vi "scaler_digital_2channel_example.vi"() -> ()   [LabVIEW 2017]
uses:
  <vilib>/Platform/TimedLoop/XDataNode/timing_clust.ctl
  <vilib>/Platform/TimedLoop/XDataNode/nitl_modes.ctl
  <vilib>/Platform/TimedLoop/XDataNode/wakeup.ctl
  <vilib>/rvi/Emulation/niFpgaGetClockAttributes.vi
  <vilib>/rvi/Emulation/niFpgaSctlEmulationGetInTimedLoop.vi
  <vilib>/rvi/Emulation/niFpgaEmulationReportErrorSimple.vi
  <vilib>/rvi/eio/common/nirviEmuTemplateMethod_errors.vi
  <vilib>/rvi/Emulation/niFpgaProcessEmulError.vi
  <vilib>/rvi/Emulation/niFpgaCriticalErrorInLSC.vi
  <vilib>/eio/EIONode/EIONode.xnode
  <vilib>/Platform/TimedLoop/XDataNode/XDataNode.xnode
  <vilib>/Platform/TimedLoop/XDataNode/XDNodeRunTimeDep.lvlib
  lib/Scaler-EPICS/scaler.lvlib
panel:
  in  "Pulse_Scaler":bool[](array[boolean])=[FALSE]
  in  "OneShot_Scaler":bool
  in  "Enable_Scaler":bool
  in  "Gate_Scaler":bool[](array[boolean])=[FALSE, FALSE]
  out "Done_Scaler":bool
  out "Counter_Scaler":u32[](array[numeric])
  in  "PresetValues_Scaler":u32[](array[numeric])=[0, 0]
  # "This is a 2 channel digital scaler. It follows to the word the definition of the scaler in the anl website\nhttps://epics.anl.gov/bcda/synApps/std/scalerRecord.html"
  # "Optimization tip:\nMake all the arrays the same size as the number\nof channels you need implemented. Setting\nthe number of channels uses up to 45% of the \nresources. Setting to 2 uses only 23%."
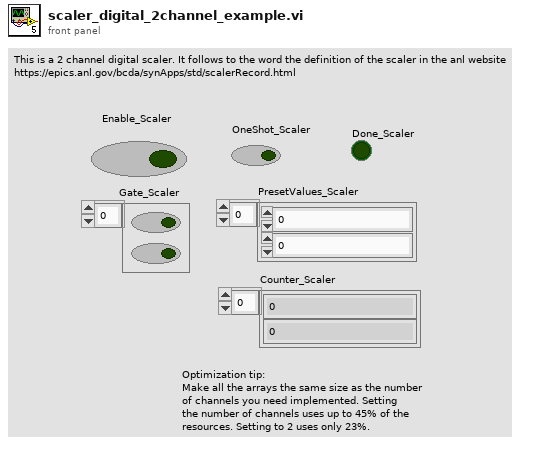
[diagram p1: front panel]
types:
  T1 = typedef "XDNodeRunTimeDep.lvlib/timing_clust.ctl" = cluster{"Expected End [f-1]":u64, "Actual End [f-1]":u64, "Finished Late? [f-1]":bool, "Expected End [i-1]":u64, "Actual End [i-1]":u64, "Finished Late? [i-1]":bool, "Expected Start [i]":u64, "Actual Start [i]":u64, "Expected Start [f]":u64, "Actual Start [f]":u64, "Source Name":string, "Structure Name":string, "Period":i64, "Deadline":i64, "Offset":i64, "Start":i64, "Priority":i32, "Timeout":i32, "Mode":T2, "Wakeup Reason":T3, "Error":errorcluster, "Source Type":string, "Secondary Source Type":string, "Global End Time":u64, "Global Start Time":u64, "Frame Duration":u64, "Iteration Duration":u64, "Assigned CPU":i32, "I/O Scan Engine Mode":u32}
  T2 = typedef "XDNodeRunTimeDep.lvlib/nitl_modes.ctl" = enum32{"No Change", "Process missed periods, maintain original phase", "Discard missed periods, maintain original phase", "Process missed periods, ignore original phase", "Discard missed periods, ignore original phase"}
  T3 = typedef "XDNodeRunTimeDep.lvlib/wakeup.ctl" = enum32{"Normal", "Aborted", "Asynchronous wakeup", "Timing source error", "Timed loop error", "Timeout"}
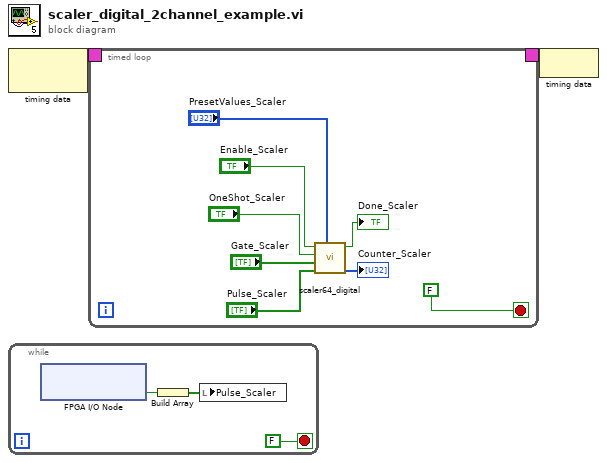
[diagram p0: block diagram]
diagram:
  n1 = node-c288() -> (w2:T1)  [unwired: 1 in]
  n2 = while {
    stop <- FALSE stop-if-true
    n3 = xnode "FPGA I/O Node"() -> ("Mod2/DIO0"=w5:bool)  [unwired: 1 in, 1 out]
    n4 = Build Array(w5) -> (w4:bool[])
    n5 = local write "Pulse_Scaler"(w4) -> ()
  }
  n6 = timed-loop {
    timing: w2 -> [_]
    timing-out: [_] -> w1
    stop <- FALSE stop-if-true
    n7 = call "scaler64_digital.vi"("PresetValues_Scaler"="PresetValues_Scaler", "Pulse_Scaler"="Pulse_Scaler", "Gate_Scaler"="Gate_Scaler", "OneShot_Scaler"="OneShot_Scaler", "Enable_Scaler"="Enable_Scaler") -> ("Counter_Scaler"=→"Counter_Scaler":u32[], "Done_Scaler"=→"Done_Scaler":bool)  [unwired: 5 in]
  }
  n8 = node-c288(w1) -> ()
